vi "Fetch Parameter Default Assignments.vi"(8 "Error In":errorcluster, 9 "Parameters":refnum<k24>[](array[refnum])) -> (0 "Error Out":errorcluster, 5 "Parameter Defaults":string[][](array[string]))   [LabVIEW 2011]
uses:
  NationalInstruments.VeriStand.RealTimeSequenceDefinitionApi
  NationalInstruments.VeriStand.DataTypes
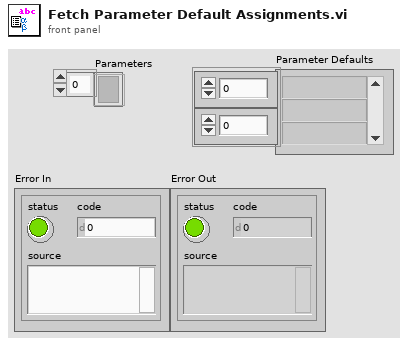
[diagram p1: front panel]
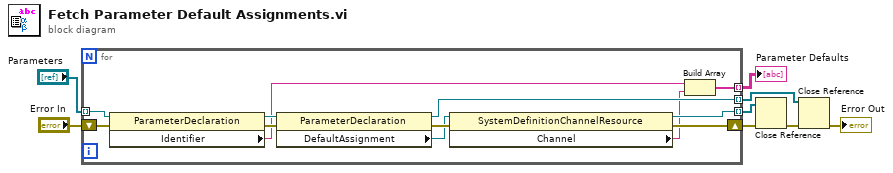
[diagram p0: block diagram]
diagram:
  n1 = for {
    tunnel: "Parameters" -> [w16] mode=indexing
    shift-right: [w14] -> w5
    shift-left: "Error In" -> [w15]
    tunnel: [w13] -> w4 mode=indexing
    tunnel: [w12] -> w2 mode=indexing
    tunnel: [w9] -> w6 mode=indexing
    n2 = property class="ParameterDeclaration"(reference=w16, error in=w15) -> (reference out=w17:refnum<k24>, error out=w18:errorcluster, "Identifier"=w11:string)
    n3 = property class="ParameterDeclaration"(reference=w17, error in=w18) -> (reference out=w12:refnum<k24>, error out=w20:errorcluster, "DefaultAssignment"=w19:refnum<k24>)
    n4 = property class="SystemDefinitionChannelResource"(reference=w19, error in=w20) -> (reference out=w13:refnum<k24>, error out=w14:errorcluster, "Channel"=w10:string)
    n5 = Build Array(w11, w10) -> (w9:string[])
  }
  "Parameter Defaults" <- w6
  n6 = Close Reference(reference=w4, error in (no error)=w5) -> (error out=w3:errorcluster)
  n7 = Close Reference(reference=w2, error in (no error)=w3) -> (error out=→"Error Out":errorcluster)
